vi "cook.vi"(8 "error in (no error)":errorcluster, 11 "PopcornPopper in":refnum<class "PopcornPopper.lvclass">) -> (0 "error out":errorcluster, 3 "PopcornPopper out":refnum<class "PopcornPopper.lvclass">)   [LabVIEW 2011, in "PopcornPopper.lvclass"]
uses:
  PopcornPopper.lvclass
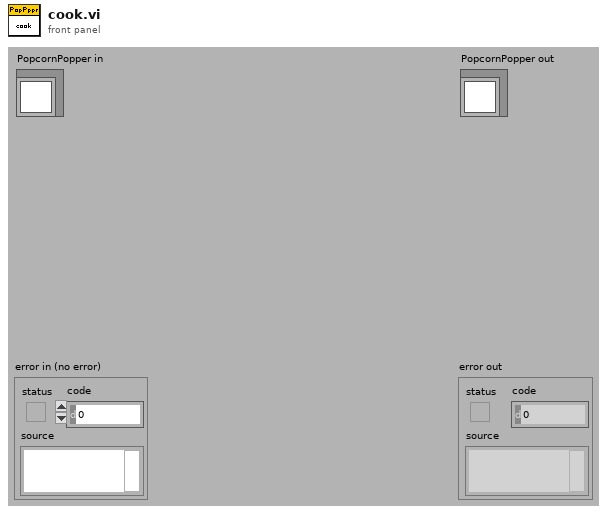
[diagram p1: front panel]
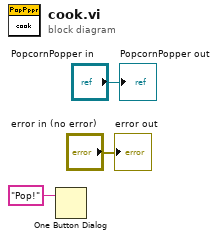
[diagram p0: block diagram]
diagram:
  n1 = One Button Dialog(message="Pop!") -> ()  [unwired: 1 in, 1 out]
  "error out" <- "error in (no error)"
  "PopcornPopper out" <- "PopcornPopper in"
